vi "GetBitfile.vi"(8 "error in (no error)":errorcluster, 9 "system info":T1, 11 "bitfile dir":path) -> (0 "error out":errorcluster, 2 "source":string, 3 "Bitfile":path, 5 "found":bool)   [LabVIEW 2017, in "CmsFpgaBitfileManager.lvlib"]
uses:
  <vilib>/addons/InsightCM/Devices/Shared/Cms/CmsFpgaBitfileManager/CmsFpgaBitfileManager.lvlib
  <vilib>/addons/cRIODetectHW/control/SystemHW.ctl
  <vilib>/addons/cRIODetectHW/control/cRIO Product Info.ctl
  <vilib>/addons/cRIODetectHW/cRIODetectHW.lvlib
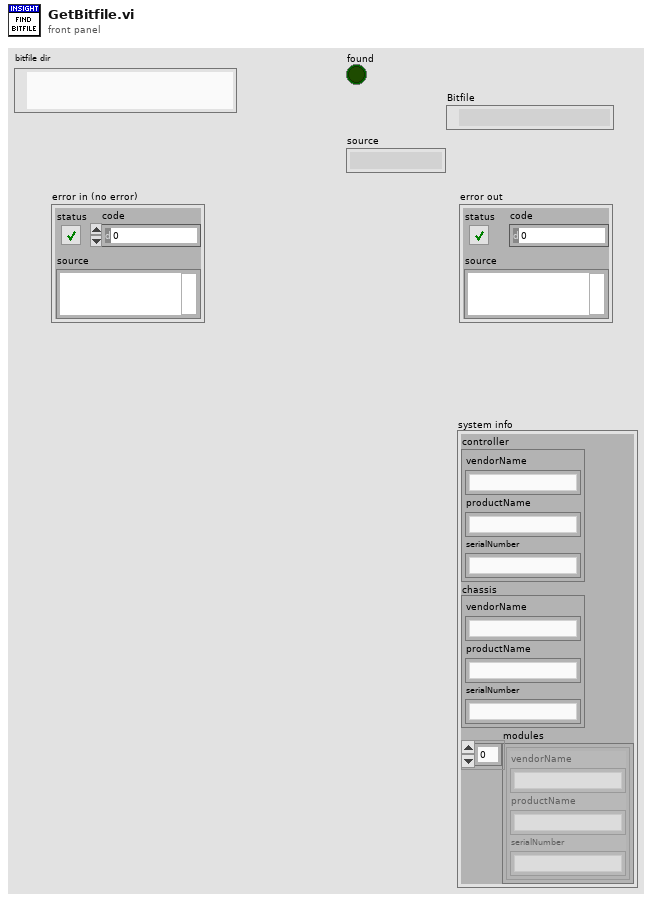
[diagram p1: front panel]
types:
  T1 = typedef "cRIODetectHW.lvlib/SystemHW.ctl" = cluster{"controller":T2, "chassis":T2, "modules":T2[]}
  T2 = typedef "cRIODetectHW.lvlib/cRIO Product Info.ctl" = cluster{"vendorName":string, "productName":string, "serialNumber":string}
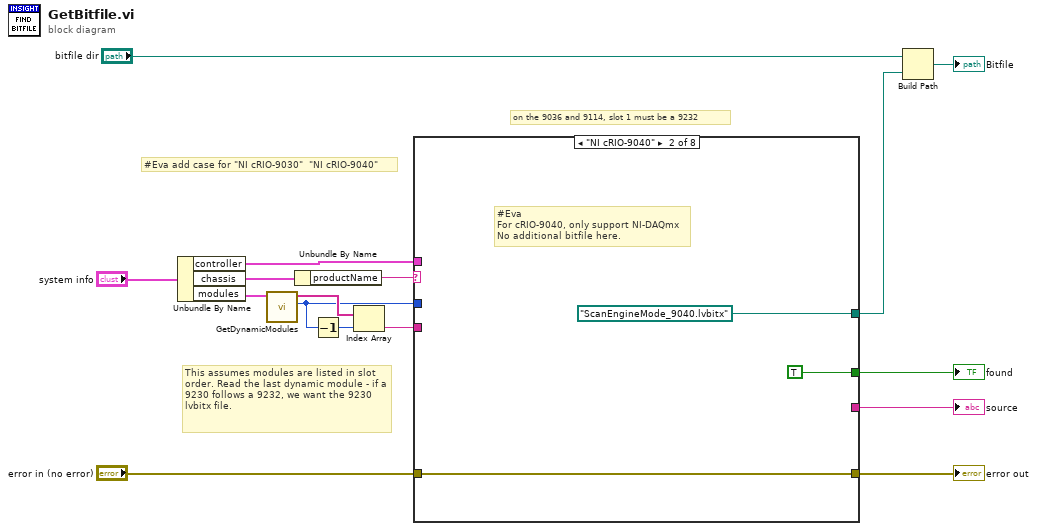
[diagram p0: block diagram]
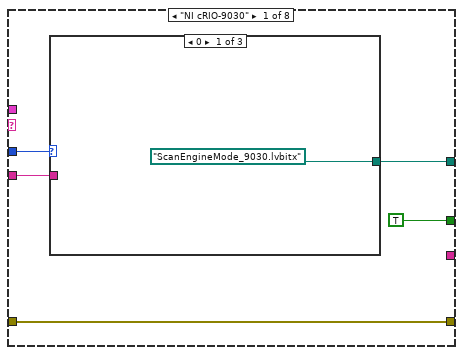
[diagram p2: hidden frame]
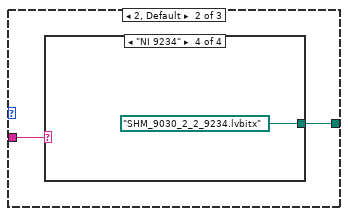
[diagram p3: hidden frame]
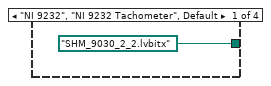
[diagram p4: hidden frame]
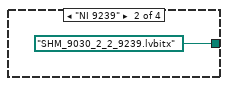
[diagram p5: hidden frame]
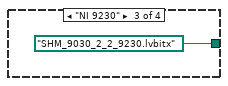
[diagram p6: hidden frame]
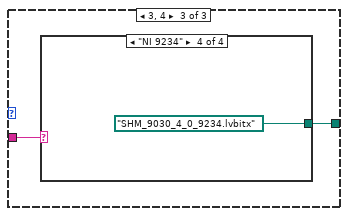
[diagram p7: hidden frame]
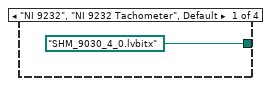
[diagram p8: hidden frame]
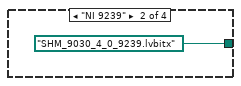
[diagram p9: hidden frame]
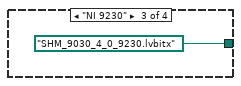
[diagram p10: hidden frame]
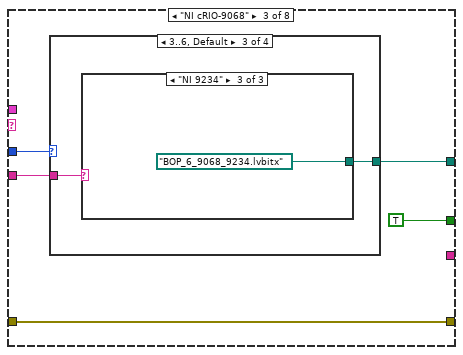
[diagram p11: hidden frame]
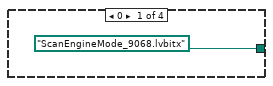
[diagram p12: hidden frame]
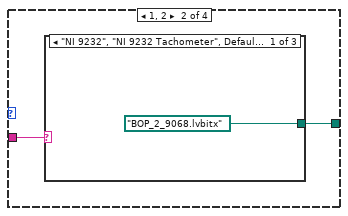
[diagram p13: hidden frame]
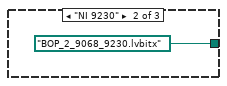
[diagram p14: hidden frame]
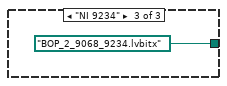
[diagram p15: hidden frame]
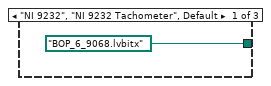
[diagram p16: hidden frame]
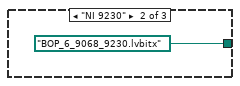
[diagram p17: hidden frame]
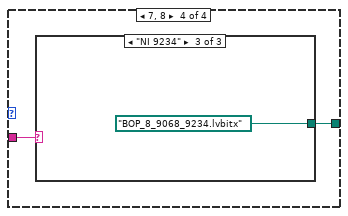
[diagram p18: hidden frame]
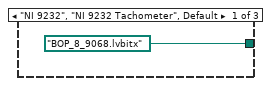
[diagram p19: hidden frame]
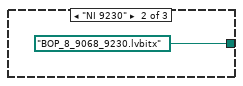
[diagram p20: hidden frame]
diagram:
  # "#Eva add case for \"NI cRIO-9030\"  \"NI cRIO-9040\""
  # "This assumes modules are listed in slot order. Read the last dynamic module - if a 9230 follows a 9232, we want the 9230 lvbitx file."
  # "on the 9036 and 9114, slot 1 must be a 9232"
  n1 = Unbundle By Name("system info") -> ("controller"=w12:T2, "chassis"=w14:T2, "modules"=w15:T2[])
  n2 = call <vilib>:"GetDynamicModules.vi"("modules"=w15) -> ("number of dynamic modules"=w7:i32, "all dynamic modules"=w9:string[])  [unwired: 8 in, 1 out]
  n3 = Unbundle By Name(w14) -> ("productName"=w13:string)
  n4 = Decrement(x=w7) -> (x-1=w6:i32)
  n5 = Index Array(array=w9, index=w6) -> (element=w8:string)
  n6 = case shown="\"NI cRIO-9040\"" w13 {
    tunnel: w12 -> [_ _ _ _ _ _ _ _]
    tunnel: w7 -> [w19 _ w40 w61 w79 _ _ _]
    tunnel: w8 -> [w20 _ w41 w62 w78 w91 w98 _]
    tunnel: [w21 path "ScanEngineMode_9040.lvbitx" w42 w63 w77 w90 w97 _] -> w4
    tunnel: [w18 w35 w39 w60 w76 w89 w96 w103] -> w11
    tunnel: "error in (no error)" -> [w18 w35 w39 w60 w76 w89 w96 w103]
    tunnel: [TRUE ("status") TRUE ("status") TRUE ("status") TRUE ("status") TRUE ("status") TRUE ("status") TRUE ("status") FALSE ("status")] -> w2
    tunnel: [_ _ _ _ _ _ _ "Unknown chassis" ("source")] -> w1
    frame "NI cRIO-9030" {
      n7 = case shown="0" w19 {
        tunnel: w20 -> [_ w23 w30]
        tunnel: [path "ScanEngineMode_9030.lvbitx" w24 w29] -> w21
        frame 0 {
        }
        frame 2, Default {
          n8 = case shown="\"NI 9234\"" w23 {
            tunnel: [path "SHM_9030_2_2.lvbitx" path "SHM_9030_2_2_9239.lvbitx" path "SHM_9030_2_2_9230.lvbitx" path "SHM_9030_2_2_9234.lvbitx"] -> w24
            frame "NI 9232", "NI 9232 Tachometer", Default {
            }
            frame "NI 9239" {
            }
            frame "NI 9230" {
            }
            frame "NI 9234" {
            }
          }
        }
        frame 3, 4 {
          n9 = case shown="\"NI 9234\"" w30 {
            tunnel: [path "SHM_9030_4_0.lvbitx" path "SHM_9030_4_0_9239.lvbitx" path "SHM_9030_4_0_9230.lvbitx" path "SHM_9030_4_0_9234.lvbitx"] -> w29
            frame "NI 9232", "NI 9232 Tachometer", Default {
            }
            frame "NI 9239" {
            }
            frame "NI 9230" {
            }
            frame "NI 9234" {
            }
          }
        }
      }
    }
    frame "NI cRIO-9040" {
      # "#Eva \nFor cRIO-9040, only support NI-DAQmx\nNo additional bitfile here."
    }
    frame "NI cRIO-9068" {
      n10 = case shown="3..6, Default" w40 {
        tunnel: w41 -> [_ w44 w50 w55]
        tunnel: [path "ScanEngineMode_9068.lvbitx" w45 w49 w54] -> w42
        frame 0 {
        }
        frame 1, 2 {
          n11 = case shown="\"NI 9232\", \"NI 9232 Tachometer\", Default" w44 {
            tunnel: [path "BOP_2_9068.lvbitx" path "BOP_2_9068_9230.lvbitx" path "BOP_2_9068_9234.lvbitx"] -> w45
            frame "NI 9232", "NI 9232 Tachometer", Default {
            }
            frame "NI 9230" {
            }
            frame "NI 9234" {
            }
          }
        }
        frame 3..6, Default {
          n12 = case shown="\"NI 9234\"" w50 {
            tunnel: [path "BOP_6_9068.lvbitx" path "BOP_6_9068_9230.lvbitx" path "BOP_6_9068_9234.lvbitx"] -> w49
            frame "NI 9232", "NI 9232 Tachometer", Default {
            }
            frame "NI 9230" {
            }
            frame "NI 9234" {
            }
          }
        }
        frame 7, 8 {
          n13 = case shown="\"NI 9234\"" w55 {
            tunnel: [path "BOP_8_9068.lvbitx" path "BOP_8_9068_9230.lvbitx" path "BOP_8_9068_9234.lvbitx"] -> w54
            frame "NI 9232", "NI 9232 Tachometer", Default {
            }
            frame "NI 9230" {
            }
            frame "NI 9234" {
            }
          }
        }
      }
    }
    frame "NI cRIO-9065" {
      n14 = case shown="3, 4" w61 {
        tunnel: w62 -> [_ w65 w71]
        tunnel: [path "ScanEngineMode_9065.lvbitx" w66 w70] -> w63
        frame 0 {
        }
        frame 2, Default {
          n15 = case shown="\"NI 9232\", \"NI 9232 Tachometer\", Default" w65 {
            tunnel: [path "CMS_9065_2_2.lvbitx" path "CMS_9065_2_2_9230.lvbitx" path "CMS_9065_2_2_9234.lvbitx"] -> w66
            frame "NI 9232", "NI 9232 Tachometer", Default {
            }
            frame "NI 9230" {
            }
            frame "NI 9234" {
            }
          }
        }
        frame 3, 4 {
          n16 = case shown="\"NI 9230\"" w71 {
            tunnel: [path "CMS_9065_4_0.lvbitx" path "CMS_9065_4_0_9230.lvbitx" path "CMS_9065_4_0_9234.lvbitx"] -> w70
            frame "NI 9232", "NI 9232 Tachometer", Default {
            }
            frame "NI 9230" {
            }
            frame "NI 9234" {
            }
          }
        }
      }
    }
    frame "NI cRIO-9114" {
      n17 = case shown="0..5" w79 {
        tunnel: w78 -> [w80 w85]
        tunnel: [w81 w84] -> w77
        frame 0..5 {
          n18 = case shown="\"NI 9230\"" w80 {
            tunnel: [path "TMS_9114.lvbitx" path "TMS_9114_9230.lvbitx"] -> w81
            frame "NI 9232", "NI 9232 Tachometer", Default {
            }
            frame "NI 9230" {
            }
          }
        }
        frame 6.., Default {
          n19 = case shown="\"NI 9232\", \"NI 9232 Tachometer\", Default" w85 {
            tunnel: [path "TMS_6Mod_9114.lvbitx" path "TMS_6Mod_9114_9230.lvbitx"] -> w84
            frame "NI 9232", "NI 9232 Tachometer", Default {
            }
            frame "NI 9230" {
            }
          }
        }
      }
    }
    frame "NI cRIO-9036" {
      n20 = case shown="\"NI 9229\"" w91 {
        tunnel: [path "CMS_9036.lvbitx" path "CMS_9036_9230.lvbitx" path "CMS_9036_9229.lvbitx"] -> w90
        frame "NI 9232", "NI 9232 Tachometer", Default {
        }
        frame "NI 9230" {
        }
        frame "NI 9229" {
        }
      }
    }
    frame "NI cRIO-9047" {
      n21 = case shown="\"NI 9232\", \"NI 9232 Tachometer\", Default" w98 {
        tunnel: [path "CMS_9047.lvbitx" path "CMS_9047_9230.lvbitx" path "CMS_9047_9229.lvbitx"] -> w97
        frame "NI 9232", "NI 9232 Tachometer", Default {
        }
        frame "NI 9230" {
        }
        frame "NI 9229" {
        }
      }
    }
    frame Default {
    }
  }
  "error out" <- w11
  "found" <- w2
  "source" <- w1
  n22 = Build Path(base path="bitfile dir", name or relative path=w4) -> (appended path=→"Bitfile":path)
